vi "HFRR ADV v04.vi"() -> ()   [LabVIEW 2025] (continued)
        tunnel: [w76 w77] -> w50
        frame False {
        }
        frame True {
          n8 = Strip Path(path=w78) -> (stripped path=w77:path)  [unwired: 1 out]
        }
      }
      n9 = Path To String(path=w50) -> (string=→"Gain path":string)
      n10 = List Folder(path=path "C:/Windows" ("directory path"), pattern="*.txt") -> (filenames=w66:string[])  [unwired: 2 in, 3 out]
      n11 = Search 1D Array(1D array=w66, element="wndcm_pw_stdED hfrr.txt") -> (index of element=w69:i32)  [unwired: 1 in]
      n12 = local write "Com flag"(u32 0 ("Com flag")) -> ()
      n13 = Equal?(x=w69, y=-1) -> (x = y?=w64:bool)
      n14 = case shown="True" w64 {
        frame False {
        }
        frame True {
          n15 = String To Byte Array(string="123\n") -> (unsigned byte array=w84:u8[])
          n16 = Array Size(array=w84) -> (size(s)=w83:i32)
          n17 = for {
            N: w83 -> [_]
            tunnel: w84 -> [w97]
            tunnel: [w94] -> w86 mode=indexing
            tunnel: w83 -> [w89]
            i -> [w87]
            n18 = Index Array(array=w97, index=w87) -> (element=w96:u8)
            n19 = Decrement(x=w89) -> (x-1=w90:i32)
            n20 = Equal?(x=w87, y=w90) -> (x = y?=w91:bool)
            n21 = Number To Decimal String(number=w96) -> (decimal integer string=w95:string)  [unwired: 1 in]
            n22 = Select(t="", s=w91, f="\r") -> (s? t:f=w88:string)
            n23 = Concatenate Strings(w95, w88) -> (w94:string)
          }
          n24 = Concatenate Strings(w86) -> (w82:string)
          n25 = local read "file path"() -> (w80:path)
          n26 = call <vilib>:"Write Characters To File.vi"("append to file? (new file:F)"=FALSE, "character string"=w82, "file path (dialog if empty)"=w80) -> ()  [unwired: 2 in, 1 out]
        }
      }
      n27 = local write "refresh flag"(FALSE ("refresh flag")) -> ()
      n28 = local write "Json End Flg"(w46) -> ()
      n29 = local write "Re-Initialise"(TRUE ("Re-Initialise")) -> ()
      n30 = local write "Upld AR 2"(TRUE ("Upld AR 2")) -> ()
      n31 = local write "Json St Flg"(w46) -> ()
      n32 = local write "FLAG 2"(0.0 ("FLAG 2")) -> ()
      n33 = local write "Lan flag"(0.0 ("Lan flag")) -> ()
      n34 = local write "Flag"(0.0 ("Flag")) -> ()
      n35 = local write "clk"(0.0 ("clk")) -> ()
      n36 = local write "COUNT"(0 ("COUNT")) -> ()
      n37 = case shown="True" "STOP" {
        frame False {
        }
        frame True {
          n38 = local write "STOP 3"(TRUE ("STOP")) -> ()
        }
      }
      n39 = local write "conststatus"(0.0 ("rpm value : 2")) -> ()
      "file path" <- path "C:/Windows/wndcm_pw_stdED hfrr.txt" ("file path")
      "FF buffer" <- dbl[] [] ("FF buffer")
    }
    frame #1 {
      n40 = Wait (ms)(milliseconds to wait=u32 1000) -> (millisecond timer value=w98:u32)
    }
    frame #2 {
      n41 = local read "Re-Initialise"() -> (w101:bool)
      n42 = case shown="True" w101 {
        frame False {
        }
        frame True {
          n43 = local write "Re-Initialise"(FALSE ("Re-Initialise")) -> ()
        }
      }
    }
  }
  n44 = local write "USER ID"(w6) -> ()
  n45 = local write "USERNAME"(w6) -> ()
  n46 = property on="Quit" class="Bool (strict)"("Value"=FALSE ("Quit")) -> (error out=w8:errorcluster)  [unwired: 2 in, 1 out]
  n47 = local write "main tab sub"(enum32{"Page 1", "Page 2"}."Page 1" ("main tab sub")) -> ()
  n48 = local write "Main Tab"(T2."HOME" ("Main Tab")) -> ()
  n49 = while {
    tunnel: w8 -> [_]
    stop <- w122 stop-if-true
    w113 = 1 ("y")
    # "New Adv Logics"
    n50 = local read "Main Tab"() -> (w120:T2)
    n51 = local read "Sign In"() -> (w109:bool)
    n52 = local read "USERNAME"() -> (w119:string)
    n53 = case shown="Default" w120 {
      frame "HOME" {
        n54 = local write "main tab sub"(enum32{"Page 1", "Page 2"}."Page 1" ("main tab sub")) -> ()
      }
      frame Default {
        n55 = local write "main tab sub"(enum32{"Page 1", "Page 2"}."Page 2" ("main tab sub")) -> ()
      }
    }
    n56 = case shown="True" w109 {
      selector: w109 -> [_ w140]
      frame False {
      }
      frame True {
        n57 = Not(x=w140) -> (.not. x?=w139:bool)
        n58 = local write "Sign In"(w139) -> ()
        n59 = local write "Main Dashboard Buttons"(T1."Dashboard" ("Main Dashboard Buttons")) -> ()
      }
    }
    n60 = local read "USER ID"() -> (w116:string)
    n61 = case shown="\"Graph Display\"" "Num/Graph" {
      frame "Numeric Display", Default {
        n62 = property on="Single/Multiple" class="RadioBtnsControl (strict)"("Visible"=FALSE) -> ()  [unwired: 2 in, 2 out]
        n63 = property on="Single - Graph" class="Ring (strict)"("Visible"=FALSE) -> ()  [unwired: 2 in, 2 out]
        n64 = local write "Main Tab Display"(T4."Dashboard 1" ("Main Tab Display")) -> ()
      }
      frame "Graph Display" {
        n65 = property on="Single/Multiple" class="RadioBtnsControl (strict)"("Visible"=TRUE) -> ()  [unwired: 2 in, 2 out]
        n66 = case shown="\"Multiple\"" "Single/Multiple" {
          frame "Single ", Default {
            n67 = property on="Single - Graph" class="Ring (strict)"("Visible"=TRUE) -> ()  [unwired: 2 in, 2 out]
            n68 = local write "Main Tab Display"(T4."Dashboard 3" ("Main Tab Display")) -> ()
          }
          frame "Multiple" {
            n69 = property on="Single - Graph" class="Ring (strict)"("Visible"=FALSE) -> ()  [unwired: 2 in, 2 out]
            n70 = local write "Main Tab Display"(T4."Dashboard 2" ("Main Tab Display")) -> ()
          }
        }
      }
    }
    n71 = call <vilib>:"Trim Whitespace.vi"("string"=w119) -> ("trimmed string"=w118:string)  [unwired: 1 in]
    n72 = call <vilib>:"Trim Whitespace.vi"("string"=w116) -> ("trimmed string"=w117:string)  [unwired: 1 in]
    n73 = String Length(string=w118) -> (length=w115:i32)
    n74 = String Length(string=w117) -> (length=w114:i32)
    n75 = case shown="\"Dashboard\"" "Main Dashboard Buttons" {
      tunnel: [T2."HOME" ("Main Tab") T2."Acquire" ("Main Tab") T2."Adv Scar" ("Main Tab") T2."Adv Scar Report" ("Main Tab") T2."Compare Files" ("Main Tab") T2."About" ("Main Tab")] -> w107
      frame "Home", Default {
      }
      frame "Dashboard" {
      }
      frame "Imaging" {
      }
      frame "Report" {
      }
      frame "Analysis" {
      }
      frame "About" {
      }
    }
    n76 = Greater?(x=w115, y=w113) -> (0:w112:bool)
    n77 = Greater?(x=w114, y=w113) -> (0:w111:bool)
    n78 = And(x=w112, y=w111) -> (x .and. y?=w110:bool)
    n79 = case shown="False" w110 {
      frame False {
        n80 = property on="Sign In" class="Bool (strict)"("DisabledEnum"=T14."Disabled" ("Disabled")) -> ()  [unwired: 2 in, 2 out]
      }
      frame True {
        n81 = property on="Sign In" class="Bool (strict)"("DisabledEnum"=T14."Enabled" ("Disabled")) -> ()  [unwired: 2 in, 2 out]
      }
    }
    n82 = Wait (ms)(milliseconds to wait=u32 100) -> ()  [unwired: 1 out]
    n83 = local write "Main Tab"(w107) -> ()
    n84 = local read "Quit"() -> (w122:bool)
    "Single" <- "Single - Graph"
  }
  n85 = while {
    stop <- w149 stop-if-true
    n86 = local read "Image Path"() -> (w147:path)
    n87 = local read "Print 3"() -> (w151:bool)
    n88 = Equal?(x=w147, y=path "") -> (x = y?=w146:bool)
    n89 = Not(x=w146) -> (.not. x?=w145:bool)
    n90 = property on="Print 3" class="Bool (strict)"("Visible"=w145) -> ()  [unwired: 2 in, 2 out]
    n91 = case shown="True" w151 {
      frame False {
        n92 = local write "Rd"(TRUE ("Boolean 7")) -> ()
      }
      frame True {
        n93 = flat-sequence {
          tunnel: [w191] -> w159
          tunnel: [w178] -> w157
          tunnel: [w188] -> w153
          tunnel: w159 -> [w200]
          tunnel: [w200] -> w158
          tunnel: w157 -> [w199]
          tunnel: [w199] -> w156
          tunnel: [w197] -> w155
          tunnel: [w196] -> w154
          tunnel: w153 -> [w196]
          tunnel: w158 -> [w202]
          tunnel: w156 -> [w203]
          tunnel: w155 -> [_]
          tunnel: w154 -> [w201]
          frame #0 {
            n94 = case shown="True" "Rd" {
              frame False {
              }
              frame True {
                n95 = while {
                  tunnel: "abcdefABCDEF" ("string 2") -> [w170]
                  shift-right: [w168] -> w162
                  shift-left: "" -> [w167]
                  i -> [w177]
                  stop <- w176 stop-if-true
                  n96 = Random Number (0-1)() -> (number: 0 to 1=w171:dbl)
                  n97 = Multiply(x=w171, y=62.0) -> (x*y=w173:dbl)
                  n98 = Decrement(x="Length 2") -> (x-1=w166:i16)
                  n99 = To Word Integer(number=w173) -> (16bit integer=w174:i16)
                  n100 = String Subset(string=w170, offset (0)=w174, length (rest)=1 ("length (rest)")) -> (substring=w169:string)
                  n101 = Greater Or Equal?(x=w177, y=w166) -> (x >= y?=w176:bool)
                  n102 = Concatenate Strings(w169, w167) -> (w168:string)
                }
                "String 10" <- w162
                n103 = local write "Rd"(FALSE ("Boolean 7")) -> ()
              }
            }
          }
          frame #1 {
            w189 = "_resized.jpg" ("command line")
            (unwired) ".jpg -resize 320x240 " ("string")
            (unwired) "Choose an Image File" ("prompt")
            # "-resize 1798x425"
            n104 = local read "Image Path"() -> (w183:path)
            n105 = Strip Path(path=w183) -> (stripped path=w178:path, name=w179:string)
            n106 = Match Pattern(string=w179, regular expression=".jpg") -> (before substring=→"before substring 2":string, after substring=→"after substring":string)  [unwired: 1 in, 2 out]
            n107 = Match Pattern(string=w179, regular expression="\\") -> (before substring=w185:string)  [unwired: 1 in, 3 out]
            n108 = Match Pattern(string=w185, regular expression=".jpg") -> (before substring=w184:string)  [unwired: 1 in, 3 out]
            n109 = Concatenate Strings("cmd /c convert " ("string"), w184, ".jpg -resize 320x240  " ("command line"), w184, w189) -> (w192:string)
            n110 = call <vilib>:"System Exec.vi"("run minimized? (F)"=TRUE, "wait until completion? (T)"=TRUE, "working directory"=w178, "command line"=w192) -> ("error out"=w191:errorcluster)  [unwired: 4 in, 3 out]
            "error out 2" <- w191
            n111 = Concatenate Strings(w184, w189) -> (w188:string)
          }
          frame #2 {
            n112 = Wait (ms)(milliseconds to wait=u32 2000 ("millisecond timer value")) -> (millisecond timer value=w197:u32)
          }
          frame #3 {
            n113 = case shown="No Error" w202 {
              tunnel: w203 -> [w206 _]
              tunnel: w201 -> [w204 _]
              frame No Error {
                (unwired) ".jpg" ("string")
                n114 = Path To String(path=w206) -> (string=w210:string)
                n115 = Concatenate Strings(w210, "\\" ("string"), w204) -> (w209:string)
                n116 = String To Path(string=w209) -> (path=w208:path)
                n117 = call <vilib>:"Read JPEG File.vi"("path to JPEG file"=w208) -> ("image data"=w212:T11)  [unwired: 8 in, 2 out]
                "image data" <- w212
                n118 = local write "Print 3"(FALSE ("Print 2")) -> ()
                n119 = call <vilib>:"Draw Flattened Pixmap.vi"("image data"=w212) -> ("new picture"=→"new picture":picture)  [unwired: 8 in]
              }
              frame Error {
              }
            }
          }
        }
      }
    }
    n120 = Wait (ms)(milliseconds to wait=u32 20 ("millisecond timer value")) -> ()  [unwired: 1 out]
    n121 = local read "EXIT"() -> (w149:bool)
  }
  n122 = disable-structure shown="Disabled" {
    disable-tunnel: [w214 _] -> w17
    disable-tunnel: w15 -> [w213 _]
    frame Disabled {
      n123 = while {
        tunnel: w213 -> [_]
        tunnel: [w216] -> w214
        tunnel: [w215] -> _
        i -> [w215]
        stop <- w216 stop-if-true
        w232 = u16 10 items=["1.0"=10, "1.5"=15, "2.0"=20] ("stop bits (10: 1 bit)")
        n124 = Wait (ms)(milliseconds to wait=u32 10) -> ()  [unwired: 1 out]
        n125 = call-poly "VISA Configure Serial Port"("VISA resource name"=refnum<visa-resource-name> "ASRL1::INSTR" ("COM PORT"), "timeout (10sec)"=u32 10, "baud rate (9600)"=u32 57600, "data bits (8)"=u16 8, "stop bits (10: 1 bit)"=w232) -> ("VISA resource name out"=w218:refnum<visa-resource-name>, "error out"=w227:errorcluster)  [unwired: 9 in]
        n126 = VISA Read(VISA resource name=w218, byte count=u32 2 ("byte count (0)")) -> (read buffer=w226:string)  [unwired: 1 in, 3 out]
        n127 = String Subset(string=w226, offset (0)=0, length (rest)=2 ("length (rest)")) -> (substring=w225:string)
        n128 = Match Pattern(string=w225, regular expression="<>") -> (offset past match=w222:i32)  [unwired: 1 in, 3 out]
        n129 = Greater Or Equal?(x=w222, y=0) -> (x >= y?=w217:bool)
        n130 = case shown="True" w217 {
          tunnel: w218 -> [_ w236]
          tunnel: w227 -> [_ w235]
          frame False {
          }
          frame True {
            n131 = VISA Read(VISA resource name=w236, byte count=u32 32 ("byte count (0)"), error in (no error)=w235) -> (read buffer=w234:string)  [unwired: 3 out]
            n132 = String Subset(string=w234, offset (0)=0, length (rest)=8 ("length (rest)")) -> (substring=w238:string)
            n133 = String Subset(string=w234, offset (0)=8, length (rest)=8 ("length (rest)")) -> (substring=w239:string)
            n134 = Decimal String To Number(string=w239) -> (number=w246:i32)  [unwired: 2 in, 1 out]
            n135 = Decimal String To Number(string=w238) -> (number=w242:i32)  [unwired: 2 in, 1 out]
            n136 = Divide(x=w246, y=10000) -> ()  [unwired: 1 out]
            n137 = Divide(x=w242, y=1000000) -> ()  [unwired: 1 out]
          }
        }
        n138 = local read "EXIT"() -> (w216:bool)
      }
    }
    frame Enabled {
    }
  }
  n139 = local write "Err Count"(0 ("Err Count")) -> ()
  n140 = local write "FRICVALZ"(0.0 ("FRICVALZ")) -> ()
  n141 = Tick Count (ms)() -> (millisecond timer value=w32:u32)
  n142 = while {
    shift-right: [w263] -> w13
    shift-left: _ -> [w253]
    shift-right: [w262] -> w12
    shift-left: errorcluster {"status"=FALSE, "code"=0, "source"="Init"} ("error out") -> [w255]
    tunnel: [w260] -> w22
    tunnel: [w261] -> _
    tunnel: w15 -> [_]
    i -> [w261]
    stop <- w260 stop-if-true
    n143 = local read "Re-Initialise"() -> (w248:bool)
    n144 = Unbundle(w255) -> ("status"=→"Port 4":bool)  [unwired: 2 out]
    n145 = flat-sequence {
      tunnel: w255 -> [w267]
      tunnel: [w267] -> w251
      frame #0 {
        n146 = Wait (ms)(milliseconds to wait=u32 50) -> ()  [unwired: 1 out]
      }
    }
    n147 = local read "Com Port 2"() -> (w254:refnum<visa-resource-name>)
    n148 = Not Equal?(x=w254, y=w253) -> (x != y?=w252:bool)
    n149 = Or(x=w252, y=w248) -> (x .or. y?=w249:bool)
    n150 = case shown="True" w249 {
      tunnel: [w264 errorcluster {"status"=TRUE, "code"=0, "source"="Init"} ("error out")] -> w250
      tunnel: w251 -> [w264 _]
      frame False {
      }
      frame True {
      }
    }
    n151 = case shown="No Error" w250 {
      selector: w250 -> [w270 w424]
      tunnel: [w272 w429] -> w263
      tunnel: [w271 w422] -> w262
      tunnel: w253 -> [w274 w427]
      tunnel: [w273 _] -> _
      frame No Error {
        n152 = stacked-sequence {
          tunnel: w274 -> [w298 _]
          tunnel: w270 -> [w297 _]
          tunnel: [w284 _] -> w273
          tunnel: [w283 _] -> w272
          tunnel: [w282 _] -> w271
          frame #0 {
            n153 = property class="Instr"(reference=w298, error in=w297) -> (reference out=w281:refnum<visa-resource-name>, error out=w296:errorcluster, "Serial Settings:Number of Bytes at Serial Port"=w277:u32)
            "Port 2" <- w277
            n154 = Greater?(x=w277, y=u32 23) -> (0:w279:bool)
            n155 = Not(x=w279) -> ()  [unwired: 1 out]
            n156 = call "Elapsed Time10"("Time Target (s)"=2.0, "Reset"=w279, "Auto Reset"=FALSE) -> ("Time has Elapsed"=→"Port 2a":bool)  [unwired: 9 in, 7 out]
            n157 = case shown="True" w279 {
              tunnel: w281 -> [w313 w338]
              tunnel: w296 -> [w312 w339]
              tunnel: [w312 w341] -> w292
              tunnel: [w313 w340] -> w293
              frame False {
              }
              frame True {
                # "Out as Volts"
                n158 = local read "Residual Due"() -> (w337:string)
                n159 = while {
                  tunnel: [w381] -> w341
                  tunnel: [w380] -> w340
                  tunnel: w339 -> [w379]
                  tunnel: w338 -> [w378]
                  tunnel: [w375] -> _
                  shift-right: [w373] -> w336
                  shift-left: w337 -> [w372]
                  i -> [w375]
                  stop <- w376 stop-if-true
                  n160 = property class="Instr"(reference=w378, error in=w379) -> (reference out=w383:refnum<visa-resource-name>, error out=w382:errorcluster, "Serial Settings:Number of Bytes at Serial Port"=w374:u32)
                  n161 = Greater?(x=w374, y=u32 8) -> (0:w376:bool)
                  n162 = VISA Read(VISA resource name=w383, byte count=w374, error in (no error)=w382) -> (VISA resource name out=w380:refnum<visa-resource-name>, read buffer=w371:string, error out=w381:errorcluster)  [unwired: 1 out]
                  n163 = Concatenate Strings(w372, w371) -> (w373:string)
                }
                n164 = while {
                  shift-right: [w364] -> w320
                  shift-left: w336 -> [w369]
                  tunnel: [w363] -> w332 mode=indexing
                  tunnel: [w362] -> _
                  i -> [w362]
                  stop <- w366 stop-if-true
                  n165 = Match Pattern(string=w369, regular expression="*") -> (after substring=w367:string)  [unwired: 1 in, 3 out]
                  n166 = Match Pattern(string=w367, regular expression="&") -> (before substring=w363:string, after substring=w364:string, offset past match=w365:i32)  [unwired: 1 in, 1 out]
                  n167 = Less Than 0?(x=w365) -> (x < 0?=w366:bool)
                }
                n168 = local write "Residual Due"(w320) -> ()
                n169 = Array Size(array=w332) -> (size(s)=w335:i32)
                n170 = Decrement(x=w335) -> (x-1=w333:i32)
                n171 = Delete From Array(array=w332, length=1, index=w333) -> (array with subset deleted=w331:string[])  [unwired: 1 out]
                n172 = Array Size(array=w331) -> (size(s)=w319:i32)
                n173 = Decrement(x=w319) -> (x-1=w318:i32)
                n174 = while {
                  tunnel: w331 -> [w350] mode=indexing
                  tunnel: w318 -> [w349]
                  tunnel: [w347] -> w326 mode=indexing
                  tunnel: [w346] -> w325 mode=indexing
                  tunnel: [w345] -> w324 mode=indexing
                  tunnel: [w344] -> w323 mode=indexing
                  tunnel: [w343] -> w321 mode=indexing
                  tunnel: [w342] -> _
                  i -> [w342]
                  stop <- w348 stop-if-true
                  w359 = u32 0 ("length (rest)")
                  w358 = ";" ("regular expression")
                  n175 = Match Pattern(string=w350, regular expression=w358) -> (before substring=w351:string, after substring=w352:string)  [unwired: 1 in, 2 out]
                  n176 = Match Pattern(string=w352, regular expression=w358) -> (before substring=w355:string, after substring=w353:string)  [unwired: 1 in, 2 out]
                  n177 = Less Or Equal?(x=w349, y=w342) -> (x <= y?=w348:bool)
                  n178 = Match Pattern(string=w353, regular expression=w358) -> (before substring=w356:string, after substring=w354:string)  [unwired: 1 in, 2 out]
                  n179 = Match Pattern(string=w354, regular expression=w358) -> (before substring=w357:string, after substring=w361:string)  [unwired: 1 in, 2 out]
                  n180 = Decimal String To Number(string=w351, default (0L)=w359) -> (number=w347:u32)  [unwired: 1 in, 1 out]
                  n181 = Decimal String To Number(string=w355, default (0L)=w359) -> (number=w346:u32)  [unwired: 1 in, 1 out]
                  n182 = Decimal String To Number(string=w356, default (0L)=w359) -> (number=w345:u32)  [unwired: 1 in, 1 out]
                  n183 = Decimal String To Number(string=w357, default (0L)=w359) -> (number=w344:u32)  [unwired: 1 in, 1 out]
                  n184 = Decimal String To Number(string=w361, default (0L)=u8 0 ("length (rest)")) -> (number=w343:u8)  [unwired: 1 in, 1 out]
                }
                "Din" <- w321
                n185 = Bundle(w326, w325, w324, w323) -> (w328:cluster{u32[], u32[], u32[], u32[]})  [unwired: 1 in]
                n186 = Divide(x=w328, y=4095 ("length (rest)")) -> (x/y=w330:cluster{dbl[], dbl[], dbl[], dbl[]})
                n187 = Multiply(x=w330, y=sgl 3.32 ("Numeric")) -> (x*y=w322:cluster{dbl[], dbl[], dbl[], dbl[]})
                n188 = Unbundle(w322) -> (→"ECR":dbl[], →"Rtemp":dbl[], →"Air temp":dbl[], →"Ch3 2":dbl[])
              }
            }
            n189 = local read "Due Com"() -> (w285:string[])
            n190 = Delete From Array(array=w285, length=1, index=0) -> (deleted portion=w288:string[], array with subset deleted=w289:string[])
            n191 = local write "Due Com"(w289) -> ()
            n192 = Index Array(array=w288, index=0) -> (element=w286:string)
            n193 = Not Equal?(x=w286, y="") -> (x != y?=w294:bool)
            n194 = case shown="True" w294 {
              tunnel: w293 -> [w300 w305]
              tunnel: [w300 w309] -> w283
              tunnel: w292 -> [w299 w304]
              tunnel: [w299 w307] -> w282
              tunnel: w286 -> [_ w303]
              tunnel: [_ w306] -> _
              frame False {
                # "DATA  WRITE LOOP"
              }
              frame True {
                n195 = Concatenate Strings(w303, "\r\n") -> (w302:string)
                n196 = VISA Write(VISA resource name=w305, write buffer=w302, error in (no error)=w304) -> (VISA resource name out=w309:refnum<visa-resource-name>, return count=w306:u32, error out=w308:errorcluster)
                n197 = flat-sequence {
                  tunnel: w308 -> [w310]
                  tunnel: [w310] -> w307
                  frame #0 {
                    n198 = Wait (ms)(milliseconds to wait=u32 5) -> ()  [unwired: 1 out]
                  }
                }
              }
            }
            n199 = Array Size(array=w285) -> (size(s)=w284:i32)
          }
          frame #1 {
            w392 = 10 ("y")
            w397 = 10 ("y")
            n200 = local read "Rtemp"() -> (w385:dbl[])
            n201 = for {
              tunnel: w385 -> [w409] mode=indexing
              shift-right: [w410] -> w393
              shift-left: dbl[] [] ("temp buf 2") -> [w411]
              n202 = Equal To 0?(x=w409) -> (x = 0?=w413:bool)
              n203 = Build Array (concatenate)(w411, w409) -> (w412:dbl[])
              n204 = Select(t=w411, s=w413, f=w412) -> (s? t:f=w410:dbl[])
            }
            n205 = local read "temp buf"() -> (w394:dbl[])
            n206 = Insert Into Array(array=w393, index=0, new element=w394) -> (w399:dbl[])
            n207 = Array Size(array=w399) -> (size(s)=w398:i32)
            n208 = Greater?(x=w398, y=w397) -> (0:w400:bool)
            n209 = case shown="True" w400 {
              tunnel: w399 -> [w414 w420]
              tunnel: w398 -> [_ w418]
              tunnel: w397 -> [_ w417]
              tunnel: [w414 w415] -> w396
              frame False {
              }
              frame True {
                n210 = Subtract(x=w418, y=w417) -> (x-y=w416:i32)
                n211 = Delete From Array(array=w420, length=w416, index=0) -> (array with subset deleted=w415:dbl[])  [unwired: 1 out]
              }
            }
            "temp buf" <- w396
            n212 = local read "ecr buf"() -> (w386:dbl[])
            n213 = local read "ECR"() -> (w384:dbl[])
            n214 = Insert Into Array(array=w384, index=0, new element=w386) -> (w390:dbl[])
            n215 = Array Size(array=w390) -> (size(s)=w391:i32)
            n216 = Greater?(x=w391, y=w392) -> (0:w389:bool)
            n217 = case shown="True" w389 {
              tunnel: w390 -> [w402 w408]
              tunnel: w391 -> [_ w406]
              tunnel: w392 -> [_ w405]
              tunnel: [w402 w403] -> w387
              frame False {
              }
              frame True {
                n218 = Subtract(x=w406, y=w405) -> (x-y=w404:i32)
                n219 = Delete From Array(array=w408, length=w404, index=0) -> (array with subset deleted=w403:dbl[])  [unwired: 1 out]
              }
            }
            "ecr buf" <- w387
          }
        }
      }
      frame Error {
        w435 = u16 0 items=["None", "XON/XOFF", "RTS/CTS", "XON/XOFF & RTS/CTS", "DTR/DSR", "XON/XOFF & DTR/DSR"] ("flow control (0:none)  2")
        w433 = u16 10 items=["1.0"=10, "1.5"=15, "2.0"=20] ("stop bits 2")
        w431 = u16 0 items=["None", "Odd", "Even", "Mark", "Space"] ("parity 2")
        w432 = u32 10000  # timeout (10sec)
        n220 = VISA Clear(VISA resource name=w427, error in (no error)=w424) -> (VISA resource name out=w426:refnum<visa-resource-name>, error out=w425:errorcluster)
        n221 = VISA Close(VISA resource name=w426, error in (no error)=w425) -> (error out=w428:errorcluster)
        n222 = local read "Com Port 2"() -> (w421:refnum<visa-resource-name>)
        "visa due" <- w421
        n223 = call <vilib>:"Clear Errors.vi"("error in (no error)"=w428) -> ()  [unwired: 5 in, 2 out]
        n224 = call-poly "VISA Configure Serial Port"("VISA resource name"=w421, "timeout (10sec)"=w432, "baud rate (9600)"=u32 250000 ("baud rate  2"), "data bits (8)"=u16 8 ("data bits  2"), "parity (0:none)"=w431, "stop bits (10: 1 bit)"=w433, "flow control (0:none)"=w435) -> ("VISA resource name out"=w436:refnum<visa-resource-name>, "error out"=w437:errorcluster)  [unwired: 7 in]
        n225 = flat-sequence {
          tunnel: w436 -> [w439]
          tunnel: w437 -> [w438]
          tunnel: [w439] -> w429
          tunnel: [w438] -> w422
          frame #0 {
            n226 = Wait (ms)(milliseconds to wait=u32 50) -> ()  [unwired: 1 out]
          }
        }
        "Residual Due" <- ""
        "Port 2 Error" <- w422
      }
    }
    n227 = local read "Port 2a"() -> (w256:bool)
    n228 = local read "Port 4"() -> (w257:bool)
    n229 = Or(x=w257, y=w256) -> (x .or. y?=w259:bool)
    n230 = case shown="True" w259 {
      frame False {
        w268 = FALSE ("Visible")
        n231 = property on="Port 2a" class="Bool (strict)"("Visible"=w268) -> ()  [unwired: 2 in, 2 out]
        n232 = property on="Port 4" class="Bool (strict)"("Visible"=w268) -> ()  [unwired: 2 in, 2 out]
      }
      frame True {
        w269 = TRUE ("Visible")
        n233 = property on="Port 2a" class="Bool (strict)"("Visible"=w269) -> ()  [unwired: 2 in, 2 out]
        n234 = property on="Port 4" class="Bool (strict)"("Visible"=w269) -> ()  [unwired: 2 in, 2 out]
      }
    }
    n235 = local read "EXIT"() -> (w260:bool)
    "Error Due" <- w255
  }
  n236 = while {
    shift-right: [w458] -> w36
    shift-left: _ -> [w446]
    shift-right: [w457] -> w35
    shift-left: errorcluster {"status"=TRUE, "code"=0, "source"="Init"} ("error IO") -> [w448]
    shift-right: [w455] -> _
    shift-left: w32 -> [w456]
    tunnel: w15 -> [_]
    tunnel: [w454] -> w23
    tunnel: [w453] -> _
    i -> [w453]
    stop <- w454 stop-if-true
    n237 = local read "Com Port 1"() -> (w447:refnum<visa-resource-name>)
    n238 = flat-sequence {
      tunnel: [w461] -> w444
      tunnel: w448 -> [w461]
      frame #0 {
        n239 = Wait (ms)(milliseconds to wait=u32 200) -> ()  [unwired: 1 out]
      }
    }
    n240 = local read "Re-Initialise"() -> (w441:bool)
    n241 = Not Equal?(x=w447, y=w446) -> (x != y?=w445:bool)
    n242 = Or(x=w445, y=w441) -> (x .or. y?=w442:bool)
    n243 = Unbundle(w448) -> ("status"=→"Port 3":bool)  [unwired: 2 out]
    n244 = case shown="True" w442 {
      tunnel: [w459 errorcluster {"status"=TRUE, "code"=0, "source"="Init"} ("error out")] -> w443
      tunnel: w444 -> [w459 _]
      frame False {
      }
      frame True {
      }
    }
    n245 = case shown="No Error" w443 {
      selector: w443 -> [w465 w791]
      tunnel: [w470 w796] -> w458
      tunnel: [w469 w788] -> w457
      tunnel: w446 -> [w468 w794]
      tunnel: w456 -> [w467 w793]
      tunnel: [w466 w793] -> w455
      frame No Error {
        n246 = stacked-sequence {
          tunnel: [w480 _ _ _ _ _] -> w470
          tunnel: [w479 _ _ _ _ _] -> w469
          tunnel: w468 -> [w475 _ _ _ _ _]
          tunnel: w465 -> [w474 _ _ _ _ _]
          tunnel: w467 -> [_ w588 _ _ _ _]
          tunnel: [_ w587 _ _ _ _] -> w466
          tunnel: [_ w559 _ _ _ _] -> _
          frame #0 {
            n247 = property class="Instr"(reference=w475, error in=w474) -> (reference out=w477:refnum<visa-resource-name>, error out=w478:errorcluster, "Serial Settings:Number of Bytes at Serial Port"=w471:u32)
            "Sps 3" <- w471
            "Port 1" <- w471
            n248 = Greater?(x=w471, y=u32 5) -> (0:w473:bool)
            n249 = Not(x=w473) -> (.not. x?=→"Port 1a":bool)
            n250 = case shown="True" w473 {
              tunnel: w477 -> [w482 w503]
              tunnel: w478 -> [w481 w504]
              tunnel: [w481 w506] -> w479
              tunnel: [w482 w505] -> w480
              frame False {
              }
              frame True {
                # "Out as Volts"
                n251 = local read "Residual Uno"() -> (w497:string)
                n252 = while {
                  tunnel: [w543] -> w506
                  tunnel: [w542] -> w505
                  tunnel: w504 -> [w541]
                  tunnel: w503 -> [w540]
                  tunnel: [w537] -> _
                  shift-right: [w533] -> w485
                  shift-left: w497 -> [w535]
                  i -> [w537]
                  stop <- w538 stop-if-true
                  n253 = property class="Instr"(reference=w540, error in=w541) -> (reference out=w545:refnum<visa-resource-name>, error out=w544:errorcluster, "Serial Settings:Number of Bytes at Serial Port"=w536:u32)
                  n254 = Greater?(x=w536, y=u32 30) -> (0:w538:bool)
                  n255 = VISA Read(VISA resource name=w545, byte count=w536, error in (no error)=w544) -> (VISA resource name out=w542:refnum<visa-resource-name>, read buffer=w534:string, error out=w543:errorcluster)  [unwired: 1 out]
                  n256 = Concatenate Strings(w535, w534) -> (w533:string)
                }
                "UnoRead" <- w485
                n257 = while {
                  shift-right: [w519] -> w496
                  shift-left: w485 -> [w525]
                  tunnel: [w518] -> w492 mode=indexing
                  tunnel: [w520] -> _
                  i -> [w520]
                  stop <- w522 stop-if-true
                  n258 = Match Pattern(string=w525, regular expression="*") -> (after substring=w523:string)  [unwired: 1 in, 3 out]
                  n259 = Match Pattern(string=w523, regular expression="&") -> (before substring=w518:string, after substring=w519:string, offset past match=w521:i32)  [unwired: 1 in, 1 out]
                  n260 = Less Than 0?(x=w521) -> (x < 0?=w522:bool)
                }
                n261 = local write "Residual Uno"(w496) -> ()
                n262 = Array Size(array=w492) -> (size(s)=w493:i32)
                n263 = Decrement(x=w493) -> (x-1=w495:i32)
                n264 = Delete From Array(array=w492, length=1, index=w495) -> (array with subset deleted=w490:string[])  [unwired: 1 out]
                n265 = Array Size(array=w490) -> (size(s)=w489:i32)
                n266 = Decrement(x=w489) -> (x-1=w488:i32)
                n267 = while {
                  tunnel: [w517] -> w501 mode=indexing
                  tunnel: [w516] -> w500 mode=indexing
                  tunnel: w490 -> [w510] mode=indexing
                  tunnel: w488 -> [w509]
                  tunnel: [w507] -> _
                  i -> [w507]
                  stop <- w508 stop-if-true
                  w511 = 0 ("length (rest)")
                  w513 = ";" ("regular expression")
                  n268 = Match Pattern(string=w510, regular expression=w513) -> (before substring=w515:string, after substring=w514:string)  [unwired: 1 in, 2 out]
                  n269 = Match Pattern(string=w514, regular expression=w513) -> (before substring=w512:string)  [unwired: 1 in, 3 out]
                  n270 = Less Or Equal?(x=w509, y=w507) -> (x <= y?=w508:bool)
                  n271 = Decimal String To Number(string=w515, default (0L)=w511) -> (number=w517:i32)  [unwired: 1 in, 1 out]
                  n272 = Decimal String To Number(string=w512, default (0L)=w511) -> (number=w516:i32)  [unwired: 1 in, 1 out]
                }
                n273 = Bundle(w501, w500) -> (w491:cluster{i32[], i32[]})  [unwired: 1 in]
                n274 = case shown="0, Default" "ADC Res" {
                  tunnel: [w528 w530] -> w484
                  frame 0, Default {
                    n275 = Divide(x=65535 ("length (rest)"), y=2 ("length (rest)")) -> (x/y=w528:dbl)
                  }
                  frame 1 {
                    n276 = Divide(x=16777216 ("length (rest)"), y=2 ("length (rest)")) -> (x/y=w530:dbl)
                  }
                }
                n277 = Divide(x=w491, y=w484) -> (x/y=w502:cluster{dbl[], dbl[]})
                n278 = Multiply(x=w502, y=sgl 5.03 ("Numeric")) -> (x*y=w499:cluster{dbl[], dbl[]})
                n279 = Unbundle(w499) -> (→"Ch1":dbl[], →"Ch0":dbl[])
              }
            }
          }
          frame #1 {
            n280 = local read "Ch1"() -> (w570:dbl[])
            n281 = call-poly <vilib>:"Mean.vi"("X"=w570) -> ("mean"=w571:dbl)  [unwired: 1 out]
            "Slide 3" <- w571
            n282 = call <vilib>:"Mean PtByPt.vi"("x"=w571, "sample length"=10, "initialize"="Reset 2") -> ("mean"=→"Mean Pos Fil 2":dbl)  [unwired: 1 in, 1 out]
            n283 = case shown="True" "Zero 2" {
              tunnel: w570 -> [_ w600]
              frame False {
              }
              frame True {
                n284 = call-poly <vilib>:"Mean.vi"("X"=w600) -> ("mean"=→"zOff 2":dbl)  [unwired: 1 out]
                n285 = local write "Zero 2"(FALSE ("Zero")) -> ()
              }
            }
            n286 = Tick Count (ms)() -> (millisecond timer value=w587:u32)
            n287 = local read "zOff 2"() -> (w580:dbl)
            n288 = Subtract(x=w587, y=w588) -> (x-y=w586:u32)
            n289 = Subtract(x=w570, y=w580) -> (x-y=w576:dbl[])
            n290 = Divide(x=w586, y=u32 1000 ("x")) -> (x/y=w584:dbl)
            n291 = Multiply(x=w576, y=1.0 ("PG Oth")) -> (x*y=w562:dbl[])
            n292 = Divide(x=w562, y=1) -> (x/y=w561:dbl[])
            "Fric Val" <- w561
            n293 = local read "FF buffer"() -> (w567:dbl[])
            n294 = call-poly <vilib>:"Mean.vi"("X"=w561) -> ("mean"=w575:dbl)  [unwired: 1 out]
            n295 = Array Size(array=w567) -> (size(s)=w569:i32)
            n296 = case shown="True" "DC corr 2" {
              tunnel: w561 -> [w603 w606]
              tunnel: [w603 w605] -> w568
              tunnel: w575 -> [_ w604]
              frame False {
              }
              frame True {
                n297 = Subtract(x=w606, y=w604) -> (x-y=w605:dbl[])
              }
            }
            n298 = Insert Into Array(array=w567, index=w569, new element=w561) -> (w564:dbl[])
            n299 = Array Size(array=w568) -> (size(s)=w583:i32)
            n300 = Array Size(array=w564) -> (size(s)=w563:i32)
            n301 = Divide(x=w583, y=w584) -> (x/y=w579:dbl)
            "Sps 2" <- w579
            n302 = Greater?(x=w563, y=1000) -> (0:w565:bool)
            n303 = Reciprocal(x=w579) -> (1/x=w577:dbl)
            "dt" <- w577
            n304 = case shown="True" w565 {
              tunnel: [w593 w596] -> w552
              tunnel: w564 -> [w593 w599]
              tunnel: w563 -> [_ w598]
              frame False {
              }
              frame True {
                n305 = Subtract(x=w598, y=1000) -> (x-y=w594:i32)
                n306 = Delete From Array(array=w599, length=w594, index=0) -> (array with subset deleted=w596:dbl[])  [unwired: 1 out]
              }
            }
            n307 = Bundle By Name("Y"=w568, "dt"=w577, "t0"=timestamp(0 s since 1904-01-01)) -> (w547:waveform(dbl))  [unwired: 1 in]
            n308 = local read "FRIC. FORCE :"() -> (w549:dbl)
            n309 = call "Elapsed Time5"("Time Target (s)"="check time s", "Reset"="Reset 3") -> ("Time has Elapsed"=w554:bool)  [unwired: 10 in, 7 out]
            n310 = Multiply(x=w549, y=21.1986) -> (x*y=w548:dbl)
            n311 = Multiply(x=w548, y=w547) -> (x*y=→"FF_Wfm":waveform(dbl))
            n312 = Negate(x=w552) -> (-x=w551:dbl[])
            n313 = local write "FF buffer"(w552) -> ()
            n314 = Array Max & Min(array=w551) -> (max value=w559:dbl)  [unwired: 3 out]
            n315 = Greater Or Equal?(x=w559, y="Threshold value") -> (x >= y?=w555:bool)
            n316 = And(x=w555, y=w554) -> (x .and. y?=w553:bool)
            n317 = case shown="True" w553 {
              frame False {
                n318 = local write "Reset 3"(FALSE ("Reset 3")) -> ()
              }
              frame True {
                n319 = local write "save dpt"(TRUE ("save dpt")) -> ()
                n320 = local write "Reset 3"(TRUE ("Reset 3")) -> ()
              }
            }
          }
          frame #2 {
            n321 = local read "FF buffer"() -> (w613:dbl[])
            n322 = Array Max & Min(array=w613) -> (max value=w608:dbl, min value=w609:dbl)  [unwired: 2 out]
            n323 = Multiply(x=1.0 ("y 2"), y="Threshold") -> ()  [unwired: 1 out]
            n324 = Subtract(x=w608, y=w609) -> (x-y=w610:dbl)
            n325 = Greater?(x=w610, y="Threshold") -> (0:w607:bool)
            n326 = case shown="True" w607 {
              tunnel: w613 -> [_ w620]
              tunnel: [_ w618] -> _
              frame False {
              }
              frame True {
                w619 = 1.0 ("y")
                n327 = Delete From Array(array=w620, length=100, index=0) -> (deleted portion=w625:dbl[])  [unwired: 1 out]
                n328 = local read "FRIC. FORCE :"() -> (w618:dbl)
                n329 = call-poly <vilib>:"Mean.vi"("X"=w625) -> ("mean"=w624:dbl)  [unwired: 1 out]
                n330 = Subtract(x=w620, y=w624) -> (x-y=w623:dbl[])
                n331 = Multiply(x=w619, y=w619) -> (x*y=w621:dbl)
                n332 = Multiply(x=w623, y=w621) -> (x*y=w622:dbl[])
                "FF cal val" <- w622
                n333 = Array Max & Min(array=w622) -> (max value=w615:dbl, min value=w614:dbl)  [unwired: 2 out]
                n334 = Array Size(array=w622) -> (size(s)=w616:i32)
                n335 = property on="FF Calibration g" class="WFGraph (strict)"("X Scale.Range:Minimum"=0.0 ("y"), "X Scale.Range:Maximum"=w616, "Y Scale.Range:Minimum"=w615, "Y Scale.Range:Maximum"=w614) -> ()  [unwired: 2 in, 2 out]
              }
            }
          }
          frame #3 {
            # "5"
            n336 = local read "Ch0"() -> (w643:dbl[])
            n337 = local read "DISPLACEMENT :"() -> (w713:dbl)
            n338 = local read "zOff 3"() -> (w716:dbl)
            n339 = Add(x=w643, y="Offset") -> (x+y=w642:dbl[])
            n340 = Subtract(x=w643, y=w716) -> (x-y=w700:dbl[])
            n341 = Multiply(x=w713, y=1.0) -> (x*y=w630:dbl)
            n342 = Multiply(x=w642, y="Gain") -> (x*y=w637:dbl[])
            "Voltage LVDT Acq" <- w637
            "gLVDTraw" <- w637
            n343 = case shown="True" "Zero 3" {
              tunnel: w643 -> [_ w731]
              frame False {
              }
              frame True {
                n344 = call-poly <vilib>:"Mean.vi"("X"=w731) -> ("mean"=→"zOff 3":dbl)  [unwired: 1 out]
                n345 = local write "Zero 3"(FALSE ("Zero")) -> ()
              }
            }
            n346 = Multiply(x=w630, y="DISPLACEMENT : 2") -> (x*y=w697:dbl)
            n347 = call-poly <vilib>:"Mean.vi"("X"=w637) -> ("mean"=w636:dbl)  [unwired: 1 out]
            n348 = Array Max & Min(array=w637) -> (max value=w641:dbl, min value=w640:dbl)  [unwired: 2 out]
            n349 = Multiply(x=w700, y=w630) -> (x*y=w712:dbl[])
            "ABS DP" <- w712
            n350 = Multiply(x=w700, y=w697) -> (x*y=w699:dbl[])
            n351 = local read "Standard Slip Gauge (mm)"() -> (w698:dbl)
            n352 = Subtract(x=w641, y=w640) -> (x-y=→"Pk-Pk":dbl)
            n353 = call-poly <vilib>:"Mean.vi"("X"=w712) -> ("mean"=w702:dbl)  [unwired: 1 out]
            n354 = call-poly <vilib>:"Mean.vi"("X"=w699) -> ("mean"=w629:dbl)  [unwired: 1 out]
            "Disp (mm)" <- w629
            "software msrnt" <- w629
            n355 = Subtract(x=w636, y="LvdtOff") -> (x-y=w635:dbl)
            n356 = case shown="True" "DC correction" {
              tunnel: w712 -> [w734 w737]
              tunnel: [w734 w736] -> w649
              tunnel: w702 -> [_ w735]
              frame False {
              }
              frame True {
                n357 = Subtract(x=w737, y=w735) -> (x-y=w736:dbl[])
              }
            }
            n358 = Threshold 1D Array(2:0.0 ("threshold y"), 3:w649) -> (0:w666:dbl)  [unwired: 1 in]
            n359 = Divide(x=w629, y=w698) -> (x/y=w696:dbl)
            n360 = Multiply(x=w696, y=w697) -> (x*y=→"DISPLACEMENT : 3":dbl)
            n361 = Equal To 0?(x=w666) -> (x = 0?=w667:bool)
            n362 = local read "dt"() -> (w715:dbl)
            n363 = case shown="True" w667 {
              tunnel: w649 -> [_ w725]
              tunnel: [w721 w722] -> w662
              tunnel: w666 -> [w721 _]
              frame False {
              }
              frame True {
                n364 = Threshold 1D Array(1:20 ("start index (0)"), 2:0.0 ("threshold y"), 3:w725) -> (0:w722:dbl)
              }
            }
            n365 = Bundle By Name("Y"=w649, "dt"=w715, "t0"=timestamp(0 s since 1904-01-01)) -> (w704:waveform(dbl))  [unwired: 1 in]
            n366 = local read "FF_Wfm"() -> (w703:waveform(dbl))
            n367 = call-poly <vilib>:"Extract Single Tone Information.vi"("time signal in"=w704) -> ("detected amplitude"=w638:dbl, "detected frequency"=→"Freq":dbl)  [unwired: 5 in, 4 out]
            n368 = Subtract(x=w635, y=w638) -> (x-y=w647:dbl)
            n369 = Add(x=w638, y=w635) -> (x+y=w646:dbl)
            n370 = Bundle(w635, w647, w646) -> (→"Slide 8":cluster{dbl, dbl, dbl})  [unwired: 1 in]
            n371 = Build Array(w704, w703) -> (w685:waveform(dbl)[])
            "Waveform Graph 2" <- w685
            n372 = Split 1D Array(array=w649, index=w662) -> (second subarray=w663:dbl[])  [unwired: 1 out]
            n373 = Index Array(array=w685) -> (element #1=w686:waveform(dbl), element #2=w688:waveform(dbl))  [unwired: 2 in]
            n374 = Multiply(x=w638, y=2.0) -> (x*y=w705:dbl)
            "Stroke" <- w705
            "Mean(RAW) Stroke" <- w705
            n375 = local read "Test \nStatus"() -> (w706:bool)
            n376 = Threshold 1D Array(1:180 ("start index (0)"), 2:0.0 ("threshold y"), 3:w663) -> (0:w661:dbl)
            n377 = Unbundle By Name(w686) -> ("Y"=w659:dbl[])
            n378 = Unbundle By Name(w688) -> ("Y"=w660:dbl[])
            n379 = Split 1D Array(array=w660, index=w662) -> (second subarray=w657:dbl[])  [unwired: 1 out]
            n380 = In Range and Coerce(upper limit=1.5, x=w705, lower limit=0.5) -> (In Range?=w709:bool)  [unwired: 1 out]
            n381 = Split 1D Array(array=w663, index=w661) -> (first subarray=w656:dbl[])  [unwired: 1 out]
            n382 = Split 1D Array(array=w657, index=w661) -> (first subarray=w654:dbl[])  [unwired: 1 out]
            n383 = Split 1D Array(array=w659, index="Window") -> (second subarray=w677:dbl[])  [unwired: 1 out]
            n384 = Not(x=w709) -> (.not. x?=w708:bool)
            n385 = And(x=w708, y=w706) -> (x .and. y?=w707:bool)
            n386 = case shown="True" w707 {
              tunnel: [i32[] [] w727] -> _
              frame False {
              }
              frame True {
                n387 = local read "Array"() -> (w730:string[])
                n388 = local read "UnoRead"() -> (w729:string)
                n389 = Build Array (concatenate)(w730, w729) -> (w728:string[])
                "Array" <- w728
                n390 = String Length(string=w728) -> (length=w727:i32[])
              }
            }
            n391 = Array Max & Min(array=w660) -> (max value=w689:dbl, min value=w690:dbl)  [unwired: 2 out]
            n392 = Array Max & Min(array=w677) -> (max value=w691:dbl, min value=w692:dbl)  [unwired: 2 out]
            n393 = call-poly <vilib>:"Hanning Window.vi"("X"=w656) -> ("Windowed X"=w655:dbl[])  [unwired: 1 out]
            n394 = call-poly <vilib>:"Hanning Window.vi"("X"=w654) -> ("Windowed X"=w653:dbl[])  [unwired: 1 out]
            n395 = Subtract(x=w691, y=w692) -> (x-y=w693:dbl)
            n396 = Subtract(x=w689, y=w690) -> (x-y=w694:dbl)
            n397 = Build Array(w655, w653) -> (→"Waveform Graph 4":dbl[][])
            n398 = local read "G_val"() -> (w679:dbl)
            n399 = Divide(x=w694, y=w693) -> (x/y=w682:dbl)
            n400 = call-poly <vilib>:"RMS.vi"("X"=w677) -> ("rms value"=w633:dbl)  [unwired: 1 out]
            "Current (A)" <- w633
            n401 = call-poly <vilib>:"RMS.vi"("X"=w654) -> ("rms value"=w678:dbl)  [unwired: 1 out]
            n402 = local read "Constant (G)"() -> (w671:dbl)
            n403 = Multiply(x=w682, y=0.2) -> (x*y=w684:dbl)
            n404 = Multiply(x=0.8 ("y"), y=w679) -> (x*y=w683:dbl)
            n405 = Divide(x=w678, y=w633) -> (x/y=w672:dbl)
            n406 = Add(x=w684, y=w683) -> (x+y=w651:dbl)
            n407 = Not A Number/Path/Refnum?(number/path/refnum=w651) -> (NaN/Path/Refnum?=w650:bool)
            n408 = Multiply(x=w672, y=0.2) -> (x*y=w673:dbl)
            n409 = Multiply(x=0.8 ("y"), y=w671) -> (x*y=w674:dbl)
            n410 = Select(t=0.0, s=w650, f=w651) -> (s? t:f=w631:dbl)
            "G_val" <- w631
            n411 = Multiply(x=w633, y=w631) -> (x*y=→"Friction Force (N)":dbl)
            n412 = Add(x=w673, y=w674) -> (x+y=w670:dbl)
            "Constant (G)" <- w670
            n413 = Bundle(w670, "t"=w631) -> (→"pk-pk":cluster{dbl, "t":dbl})  [unwired: 1 in]
          }
          frame #4 {
            # "C:\\WinDucom\\data\\"
            # "?C:\\LAB-IQ-NXT\\data"
            n414 = case shown="True" "save dpt" {
              frame False {
              }
              frame True {
                n415 = local read "FF buffer"() -> (w749:dbl[])
                n416 = local read "ABS DP"() -> (w748:dbl[])
                n417 = Build Array(w749, w748) -> (w744:dbl[][])
                n418 = Transpose 2D Array(2D array=w744) -> (transposed array=w743:dbl[][])
